vi "Set Value.vi"(6 "Data":variant, 8 "error in (no error)":errorcluster, 9 "Target":i64, 10 "Target (String)":string, 11 "Hardware Interface in":refnum<class "Hardware Interface.lvclass">) -> (0 "error out":errorcluster, 3 "Hardware Interface out":refnum<class "Hardware Interface.lvclass">)   [LabVIEW 2022 SP3, in "Hardware Interface.lvclass"]
uses:
  Hardware Interface.lvclass
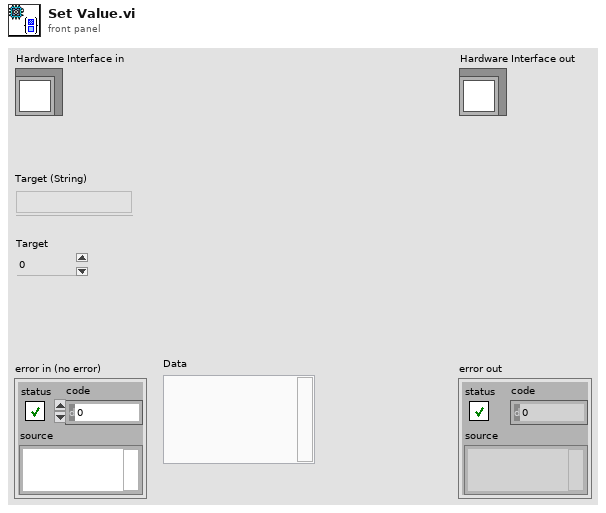
[diagram p1: front panel]
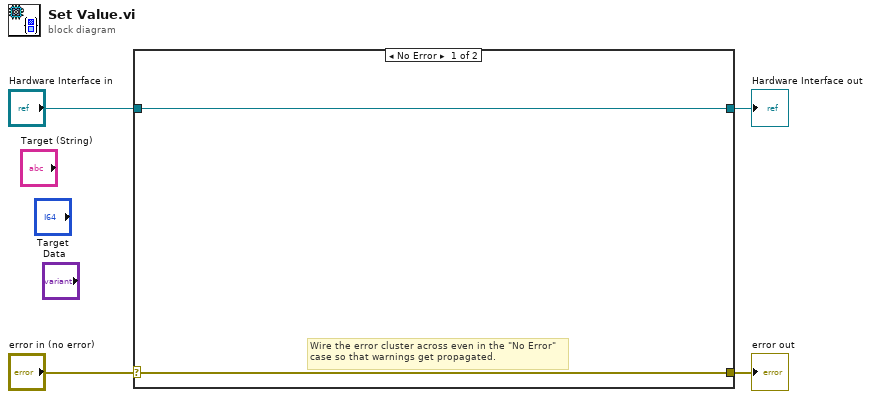
[diagram p0: block diagram]
diagram:
  n1 = case shown="No Error" "error in (no error)" {
    selector: "error in (no error)" -> [w5 w8]
    tunnel: [w5 w8] -> w3
    tunnel: [w6 w7] -> w1
    tunnel: "Hardware Interface in" -> [w6 w7]
    frame No Error {
      # "Wire the error cluster across even in the \"No Error\"\ncase so that warnings get propagated."
    }
    frame Error {
    }
  }
  "error out" <- w3
  "Hardware Interface out" <- w1
